vi "ResMgr-StartWatchDog.vi"(6 "Force?":bool, 8 "error in (no error)":errorcluster, 11 "ModuleName":string) -> (0 "error out":errorcluster, 3 "WatchDogQ":refnum<queue>)   [LabVIEW 2017, in "Communicable State Machine.lvlib"]
uses:
  Communicable State Machine.lvlib
  ResMgr-WatchdogThread.vi
  _Shared/CSM Shared.lvlib
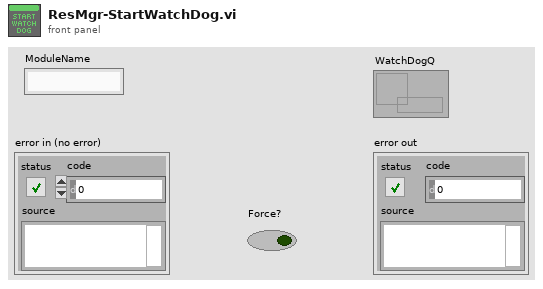
[diagram p1: front panel]
types:
  T1 = cluster{"ResType":string, "RespQ":refnum<queue>, "Parameter":string, "WatchDogQ":refnum<queue>}
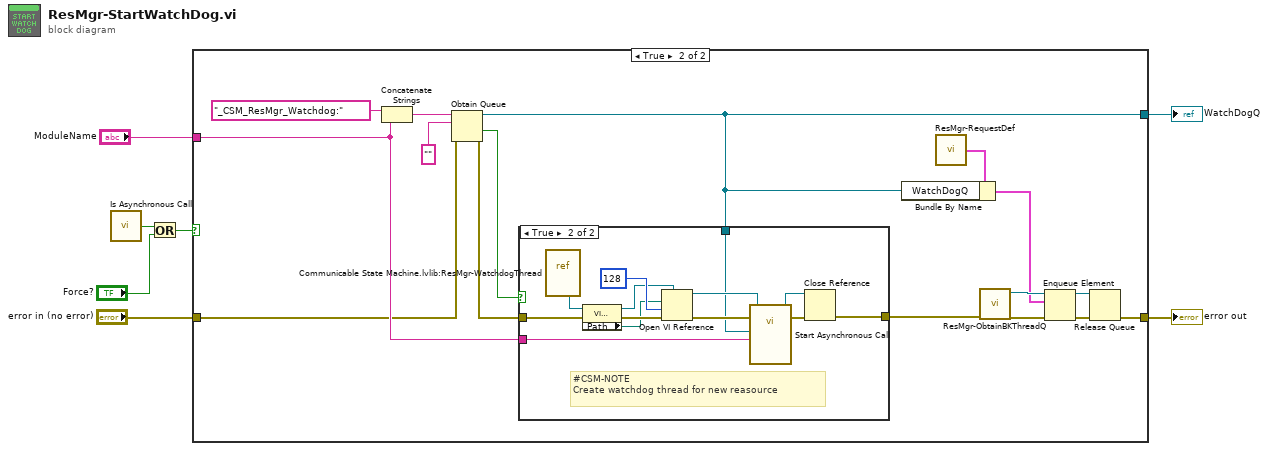
[diagram p0: block diagram]
diagram:
  n1 = call "Is Asynchronous Call.vi"() -> ("Async Call?"=w2:bool)  [unwired: 1 in]
  n2 = Or(x=w2, y="Force?") -> (x .or. y?=w3:bool)
  n3 = case shown="True" w3 {
    tunnel: "error in (no error)" -> [w8 w12]
    tunnel: "ModuleName" -> [_ w13]
    tunnel: [_ w16] -> w5
    tunnel: [w8 w14] -> w4
    frame False {
    }
    frame True {
      n4 = Concatenate Strings("_CSM_ResMgr_Watchdog:" ("string"), w13) -> (w22:string)
      n5 = Obtain Queue(name (unnamed)=w22, element data type="" ("string"), error in (no error)=w12) -> (queue out=w16:refnum<queue>, created new?=w9:bool, error out=w11:errorcluster)  [unwired: 2 in]
      n6 = case shown="True" w9 {
        tunnel: w16 -> [_ w29]
        tunnel: [w25 w28] -> w15
        tunnel: w13 -> [_ w27]
        tunnel: w11 -> [w25 w26]
        frame False {
        }
        frame True {
          # "#CSM-NOTE\nCreate watchdog thread for new reasource"
          n7 = vi-ref "Communicable State Machine.lvlib:ResMgr-WatchdogThread.vi"() -> (w31:refnum<vi>)
          n8 = property class="VI (strict)"(reference=w31, error in=w26) -> (reference out=w35:refnum<vi>, error out=w33:errorcluster, "Path"=w32:path)
          n9 = Open VI Reference(type specifier VI Refnum (for type only)=w35, vi path=w32, options=128, error in (no error)=w33) -> (vi reference=w34:refnum<vi>, error out=w30:errorcluster)  [unwired: 2 in]
          n10 = call-by-ref "Start Asynchronous Call"(reference=w34, error in=w30, "From Who"=w27, "WatchDogQ"=w29) -> (reference out=w37:refnum<vi>, error out=w36:errorcluster)  [unwired: 10 in]
          n11 = Close Reference(reference=w37, error in (no error)=w36) -> (error out=w28:errorcluster)
        }
      }
      n12 = call "ResMgr-RequestDef.vi"() -> ("ResMgr-RequestDef.ctl"=w10:T1)  [unwired: 2 in]
      n13 = Bundle By Name(cluster=w10, "WatchDogQ"=w16) -> (w17:T1)
      n14 = call "ResMgr-ObtainBKThreadQ.vi"("error in (no error)"=w15) -> ("error out"=w20:errorcluster, "ObtainBKThreadQ"=w21:refnum<queue>)  [unwired: 9 in]
      n15 = Enqueue Element(queue=w21, element=w17, error in (no error)=w20) -> (queue out=w19:refnum<queue>, error out=w18:errorcluster)  [unwired: 1 in, 1 out]
      n16 = Release Queue(queue=w19, error in (no error)=w18) -> (error out=w14:errorcluster)  [unwired: 1 in, 2 out]
    }
  }
  "WatchDogQ" <- w5
  "error out" <- w4
